vi "TestTemperature.vi"() -> ()   [LabVIEW 2018]
uses:
  <instrlib>/Mercury iXX/Public/Controls/Unit String.ctl
  <instrlib>/Mercury iXX/Public/Controls/Comms Transport Layer.ctl
  <instrlib>/Mercury iXX/Public/Libraries/System/Open/Open System.vi
  <instrlib>/Mercury iXX/Public/Libraries/System/Read/Catalogue (Read).vi
  <instrlib>/Mercury iXX/Public/Libraries/Temperature/Open/Open Temperature Device.vi
  <instrlib>/Mercury iXX/Public/Libraries/Temperature/Signals/Read/Temperature (Read).vi
  <instrlib>/Mercury iXX/Mercury iXX.lvlib
  <instrlib>/Mercury iXX/Public/Libraries/System.lvlib
  <instrlib>/Mercury iXX/Public/Libraries/Temperature.lvlib
panel:
  out "Temperature (Cryostat)":dbl
  out "Unit (Cryostat)":T1
  out "Temperature (Cell)":dbl
  out "Unit (Cell)":T1
  in  "Stop Data Collection":bool
  in  "Read Interval (s)":sgl=1.0 min=0.25 max=1000 step=0.25 format="%.2f"
  out "Mercury Error":errorcluster
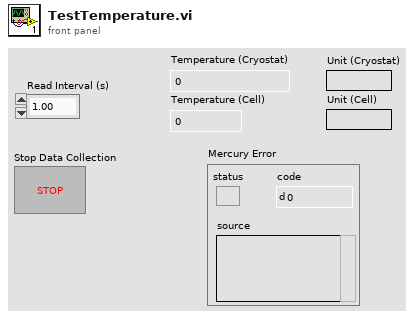
[diagram p1: front panel]
types:
  T1 = typedef "Mercury iXX.lvlib/Unit String.ctl" = string
  T2 = typedef "Mercury iXX.lvlib/Comms Transport Layer.ctl" = enum16{"Ethernet TCP/IP", "USB", "ISOBus - RS-232", "GPIB"}
  T3 = typedef "Mercury iXX.lvlib/Mercury Reference.ctl" = cluster{"Comms":refnum<visa-resource-name>, "Device ID":string[], "Comms Layer":T2, "Command":string, "Query reference":T4}
  T4 = typedef "Mercury iXX.lvlib/Query Dynamic Reference.ctl" = refnum<vi>
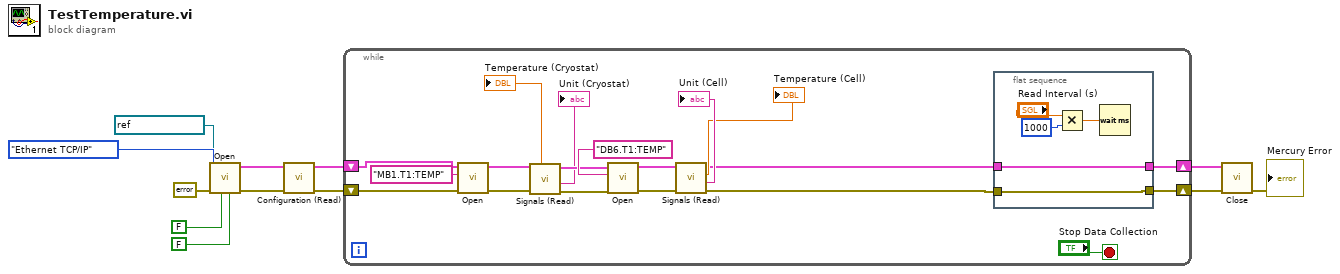
[diagram p0: block diagram]
diagram:
  n1 = call-poly <instrlib>:"Open.vi"("Clear Previous Connections (False)"=FALSE, "ID Query (True)"=FALSE, "error in (no error)"=errorcluster {"status"=FALSE, "code"=0, "source"=""}, "Comms Layer"=Comms_Transport_Layer."Ethernet TCP/IP", "VISA resource name"=refnum<visa-resource-name> "MercuryiTC") -> ("error out"=w11:errorcluster, "Mercury Reference Out"=w12:T3)  [unwired: 2 in, 3 out]
  n2 = call-poly <instrlib>:"Configuration (Read).vi"("error in"=w11, "Mercury Reference In"=w12) -> ("error out"=w5:errorcluster, "Mercury Reference Out"=w4:T3)  [unwired: 6 in, 2 out]
  n3 = while {
    shift-right: [w27] -> w10
    shift-left: w5 -> [w22]
    shift-right: [w25] -> w9
    shift-left: w4 -> [w21]
    stop <- "Stop Data Collection" stop-if-true
    n4 = call-poly <instrlib>:"Open.vi"("error in (no error)"=w22, "Device Identifier"="MB1.T1:TEMP", "Mercury Reference In"=w21) -> ("error out"=w17:errorcluster, "Mercury Reference Out"=w18:T3)  [unwired: 7 in]
    n5 = call-poly <instrlib>:"Signals (Read).vi"("error in"=w17, "Mercury Reference In"=w18) -> ("error out"=w16:errorcluster, "Unit"=→"Unit (Cryostat)":T1, "Temperature"=→"Temperature (Cryostat)":dbl, "Mercury Reference Out"=w15:T3)  [unwired: 5 in, 1 out]
    n6 = call-poly <instrlib>:"Open.vi"("error in (no error)"=w16, "Device Identifier"="DB6.T1:TEMP", "Mercury Reference In"=w15) -> ("error out"=w20:errorcluster, "Mercury Reference Out"=w19:T3)  [unwired: 7 in]
    n7 = call-poly <instrlib>:"Signals (Read).vi"("error in"=w20, "Mercury Reference In"=w19) -> ("error out"=w28:errorcluster, "Unit"=→"Unit (Cell)":T1, "Temperature"=→"Temperature (Cell)":dbl, "Mercury Reference Out"=w26:T3)  [unwired: 5 in, 1 out]
    n8 = flat-sequence {
      tunnel: w28 -> [w33]
      tunnel: [w33] -> w27
      tunnel: w26 -> [w32]
      tunnel: [w32] -> w25
      frame #0 {
        n9 = Multiply(x="Read Interval (s)", y=u32 1000 ("millisecond multiple")) -> (x*y=w34:sgl)
        n10 = Wait (ms)(milliseconds to wait=w34) -> ()  [unwired: 1 out]
      }
    }
  }
  n11 = call <instrlib>:"Close.vi"("error in (no error)"=w10, "Mercury Reference"=w9) -> ("error out"=→"Mercury Error":errorcluster)  [unwired: 9 in]
